vi "Is Empty.vi"(7 "array in":T1) -> (2 "empty?":bool, 3 "array out":T1)   [LabVIEW 2009, in "Tools_KeyedArray.lvlib"]
doc: "Adds a new element identified by <B>key</B> and containing <B>value</B> to <B>array in</B>."
uses:
  Tools_KeyedArray.lvlib
  KeyedArray.ctl
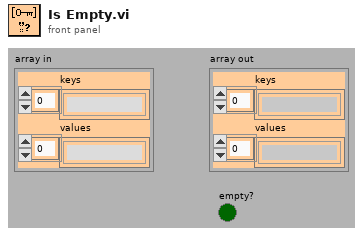
[diagram p1: front panel]
types:
  T1 = typedef "Tools_KeyedArray.lvlib/KeyedArray.ctl" = cluster{"keys":string[], "values":string[]}
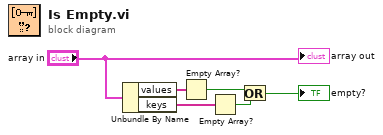
[diagram p0: block diagram]
diagram:
  n1 = Unbundle By Name("array in") -> ("values"=w5:string[], "keys"=w4:string[])
  n2 = Empty Array?(array=w5) -> (empty?=w2:bool)
  n3 = Empty Array?(array=w4) -> (empty?=w3:bool)
  n4 = Or(x=w2, y=w3) -> (x .or. y?=→"empty?":bool)
  "array out" <- "array in"
